vi "Move.vi"(8 "error in (no error)":errorcluster, 9 "Absolute (T)":bool=TRUE, 10 "Point":refnum<class "Point.lvclass">, 11 "Collection in":refnum<class "Collection.lvclass">) -> (0 "error out":errorcluster, 3 "Collection out":refnum<class "Collection.lvclass">)   [LabVIEW 2021, in "Picture2D.lvlib" / "Collection.lvclass"]
uses:
  Collection.lvclass
  IDrawable/IDrawable.lvclass
  Point/Point.lvclass
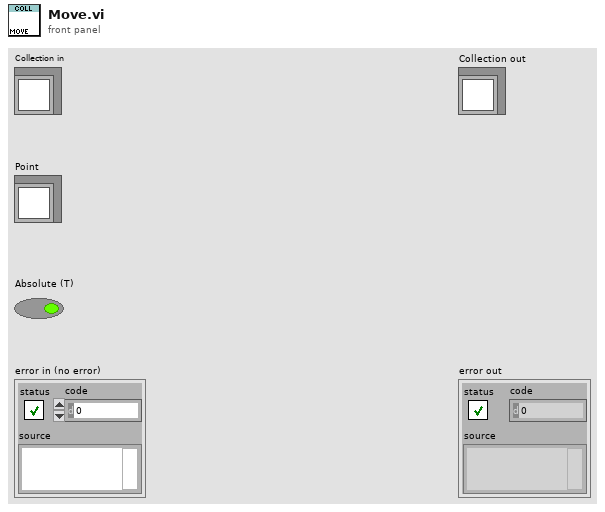
[diagram p1: front panel]
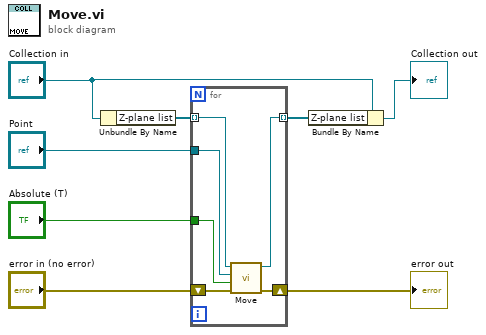
[diagram p0: block diagram]
diagram:
  n1 = Unbundle By Name("Collection in") -> ("Z-plane list"=w3:refnum<class "IDrawable.lvclass">[])
  n2 = for {
    tunnel: "Point" -> [w14]
    tunnel: "Absolute (T)" -> [w13]
    shift-right: [w11] -> w4
    shift-left: "error in (no error)" -> [w12]
    tunnel: w3 -> [w10] mode=indexing
    tunnel: [w9] -> w1 mode=indexing
    n3 = call-dynamic "Move.vi"("error in (no error)"=w12, "Absolute (T)"=w13, "Point"=w14, "IMovable in"=w10) -> ("error out"=w11:errorcluster, "IMovable out"=w9:refnum<class "IDrawable.lvclass">)  [unwired: 6 in]
  }
  "error out" <- w4
  n4 = Bundle By Name(cluster="Collection in", "Z-plane list"=w1) -> (→"Collection out":refnum<class "Collection.lvclass">)
